vi "Draw Point new.vi"(0 "picture":picture, 2 "point(x,y)":cluster{"x":i16, "y":i16}, 4 "color(black)":u32(colorbox), 8 "pen":T1={"Width"=1, "Style"=enum."Solid"}) -> (6 "new picture":picture)   [LabVIEW 2012]
doc: "Sets a pixel in a picture to a specified color."
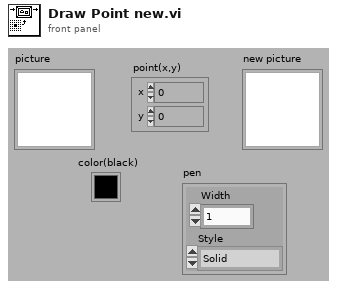
[diagram p1: front panel]
types:
  T1 = cluster{"Width":u16, "Style":enum32{"Solid", "Dash", "Dot", "DashDot", "DashDotDot"}}
  T2 = cluster{"opcode-Set Pixel":i16, "size":i32, cluster{"y":i16, "x":i16}}
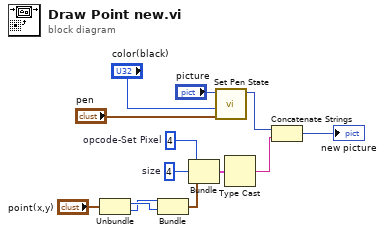
[diagram p0: block diagram]
diagram:
  w13 = i16 4  # opcode-Set Pixel
  w12 = 4  # size
  n1 = Unbundle("point(x,y)") -> ("x"=w8:i16, "y"=w7:i16)
  n2 = Bundle("y"=w7, "x"=w8) -> (w6:cluster{"y":i16, "x":i16})  [unwired: 1 in]
  n3 = Bundle("opcode-Set Pixel"=w13, "size"=w12, w6) -> (w10:T2)  [unwired: 1 in]
  n4 = call <vilib>:"Set Pen State.vi"("pen"="pen", "color(black)"="color(black)", "Picture"="picture") -> ("Picture 2"=w5:picture)  [unwired: 6 in]
  n5 = Type Cast(x=w10) -> (*(type *) &x=w9:string)  [unwired: 1 in]
  n6 = Concatenate Strings(w5, w9) -> (→"new picture":picture)
